vi "Reset.vi"(8 "error in (no error)":errorcluster, 10 "Message in":refnum<class "ResetMessage.lvclass">, 11 "DAQOrcaFlash in":refnum<class "DAQOrcaFlash.lvclass">) -> (0 "error out":errorcluster, 3 "DAQOrcaFlash out":refnum<class "DAQOrcaFlash.lvclass">)   [LabVIEW 2012, in "DAQOrcaFlash.lvclass"]
doc: "The reset method processes the command 'reset'. \n\nResets the internal state of the component (without performing a full initialisation). This could be resetting hardware, or private data to default values."
uses:
  DAQOrcaFlash.lvclass
  <vilib>/Distrio/Murmex/ResetMessage/ResetMessage.lvclass
  <vilib>/Distrio/Murmex/InitialiseMessage/InitialiseMessage.lvclass
  <vilib>/Distrio/Murmex/StopMessage/StopMessage.lvclass
  <vilib>/Utility/sysdir.llb/System Directory Type.ctl
  <vilib>/Distrio/Murmex/Murmex/Murmex.lvclass
  <vilib>/Utility/file.llb/Write To Spreadsheet File (DBL).vi
panel:
  # "This method is called when the RESET\ntrigger is sent. \n\nOverride this method when your component needs to\nrespond to this trigger. \n\nCall parent for proper implementation"
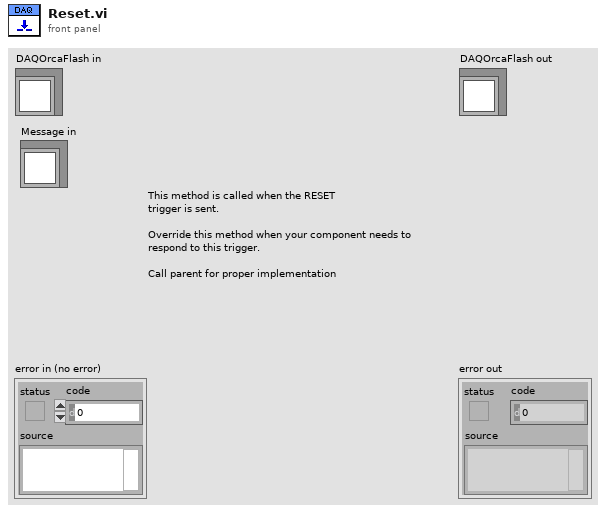
[diagram p1: front panel]
types:
  T1 = typedef "System Directory Type.ctl" = i32
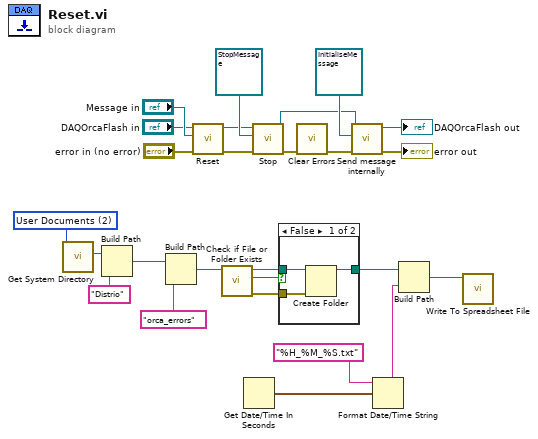
[diagram p0: block diagram]
diagram:
  w11 = T1 2 items=["User Home"=0, "User Desktop"=1, "User Documents"=2, "User Application Data"=3, "User Preferences"=4, "User Temporary"=5, "Public Documents"=6, "Public Application Data"=7, "Public Preferences"=8, "Public Cache"=13, "System Core Libraries"=9, "System Installed Libraries"=10, "Application Files"=11, "Boot Volume Root"=12] ("system directory type")
  n1 = call <vilib>:"Get System Directory.vi"("system directory type"=w11) -> ("system directory"=w10:path)  [unwired: 10 in]
  n2 = Build Path(base path=w10, name or relative path="Distrio") -> (appended path=w8:path)
  n3 = Build Path(base path=w8, name or relative path="orca_errors") -> (appended path=w4:path)
  n4 = call-parent "Reset.vi"("error in (no error)"="error in (no error)", "Message in"="Message in", "Murmex in"="DAQOrcaFlash in") -> ("error out"=w19:errorcluster, "Murmex out"=w17:refnum<class "DAQOrcaFlash.lvclass">)  [unwired: 7 in]
  n5 = call <vilib>:"Check if File or Folder Exists.vi"("path"=w4) -> ("error out"=w2:errorcluster, "file or folder exists?"=w1:bool, "dup path"=w5:path)  [unwired: 8 in]
  n6 = Get Date/Time In Seconds() -> (seconds since 1Jan1904=w14:timestamp)
  n7 = call-dynamic "Stop.vi"("error in (no error)"=w19, "Message in"=refnum<class "StopMessage.lvclass"> refnum, "DAQMH121119OrcaFlash in"=w17) -> ("error out"=w18:errorcluster, "DAQMH121119OrcaFlash out"=w16:refnum<class "DAQOrcaFlash.lvclass">)  [unwired: 7 in]
  n8 = case shown="False" w1 {
    tunnel: w5 -> [w29 w30]
    tunnel: [w28 w30] -> w3
    tunnel: w2 -> [w27 _]
    frame False {
      n9 = Create Folder(path (use dialog)=w29, error in=w27) -> (created path=w28:path)  [unwired: 1 in, 2 out]
    }
    frame True {
    }
  }
  n10 = call <vilib>:"Clear Errors.vi"("error in (no error)"=w18) -> ("error out"=w15:errorcluster)  [unwired: 6 in]
  n11 = call <vilib>:"Send message internally.vi"("error in (no error)"=w15, "Message"=refnum<class "InitialiseMessage.lvclass"> refnum ("Message in"), "Murmex in"=w16) -> ("error out"=→"error out":errorcluster, "Murmex out"=→"DAQOrcaFlash out":refnum<class "DAQOrcaFlash.lvclass">)  [unwired: 7 in]
  n12 = Format Date/Time String(time format string (%c)="%H_%M_%S.txt", seconds (now)=w14) -> (date/time string=w7:string)  [unwired: 1 in]
  n13 = Build Path(base path=w3, name or relative path=w7) -> (appended path=w6:path)
  n14 = call-poly <vilib>:"Write To Spreadsheet File.vi"("file path (dialog if empty)"=w6) -> ()  [unwired: 7 in, 1 out]
